vi "Get Self Queue.vi"(11 "Actor in":refnum<class "Actor.lvclass">) -> (2 "Self Queue":refnum<class "Priority Message Queue.lvclass">, 3 "Actor out":refnum<class "Actor.lvclass">)   [LabVIEW 2020, in "Artifex.lvlib" / "Actor.lvclass"]
uses:
  Actor.lvclass
  Actor Proxy/Actor API.lvclass
  Priority Message Queue/Priority Message Queue.lvclass
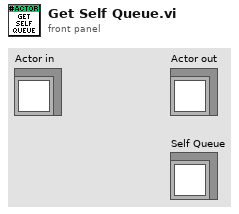
[diagram p1: front panel]
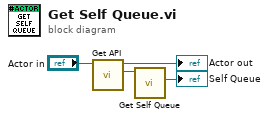
[diagram p0: block diagram]
diagram:
  n1 = call-dynamic "Get API.vi"("Actor in"="Actor in") -> ("Actor API"=w3:refnum<class "Actor API.lvclass">, "Actor out"=→"Actor out":refnum<class "Actor.lvclass">)  [unwired: 8 in, 1 out]
  n2 = call "Get Self Queue.vi"("Actor API in"=w3) -> ("Self Queue"=→"Self Queue":refnum<class "Priority Message Queue.lvclass">)  [unwired: 8 in, 2 out]
